vi "niRFUtil CONV DBL to I64.vi"(7 "Numeric (DBL)":dbl format="%#_13g") -> (8 "Numeric (I64)":i64)   [LabVIEW 2015, in "niRFUtil.lvlib"]
uses:
  niRFUtil.lvlib
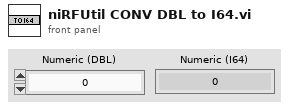
[diagram p1: front panel]
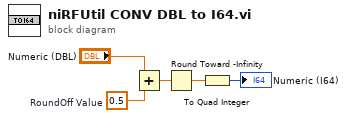
[diagram p0: block diagram]
diagram:
  w5 = 0.5  # RoundOff Value
  n1 = Add(x="Numeric (DBL)", y=w5) -> (x+y=w4:dbl)
  n2 = Round Toward -Infinity(1:w4) -> (0:w3:dbl)
  n3 = To Quad Integer(1:w3) -> (0:→"Numeric (I64)":i64)
